vi "Pull Data For Data and Queue for DB.vi"(7 "Weather Data queue":refnum<queue>, 8 "error in (no error)":errorcluster, 9 "Airport Code":string, 10 "Time Stamp":timestamp, 11 "Refnum in":T1) -> (0 "error out":errorcluster, 3 "Refnum out":T1)   [LabVIEW 2012]
uses:
  <vilib>/httpClient/ClientHandle.ctl
  TypeDef/WeatherData.ctl
  GUI Helpers/Status Helper Action.ctl
  <vilib>/httpClient/LabVIEWHTTPClient.lvlib
panel:
  out "body":string
  out "headers":string
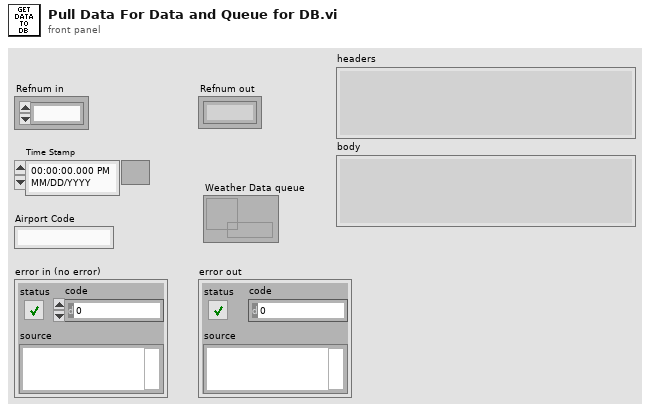
[diagram p1: front panel]
types:
  T1 = typedef "LabVIEWHTTPClient.lvlib/ClientHandle.ctl" = refnum<k1>
  T2 = typedef "Status Helper Action.ctl" = enum16{"Init", "Load Number Of Days", "Inc Add to Queue ", "Inc Get HTTP Data", "Add Push to DB", "Inc Push To DB", "Read"}
  T3 = typedef "LVDateTimeRec.ctl" = cluster{"fractional second":dbl, "second":i32, "minute":i32, "hour":i32, "day of month":i32, "month":i32, "year":i32, "day of week":i32, "day of year":i32, "DST":i32}
  T4 = typedef "WeatherData.ctl" = cluster{"TimeEST":timestamp, "TemperatureF":dbl, "DewPointF":dbl, "Humidity":i32, "Sea Level PressureIn":dbl, "VisibilityMPH":dbl, "Wind Direction":string, "Wind SpeedMPH":dbl, "Gust SpeedMPH":dbl, "PrecipitationIn":dbl, "Events":string, "Conditions":string, "WindDirDegrees":i32, "datetimeest":timestamp}
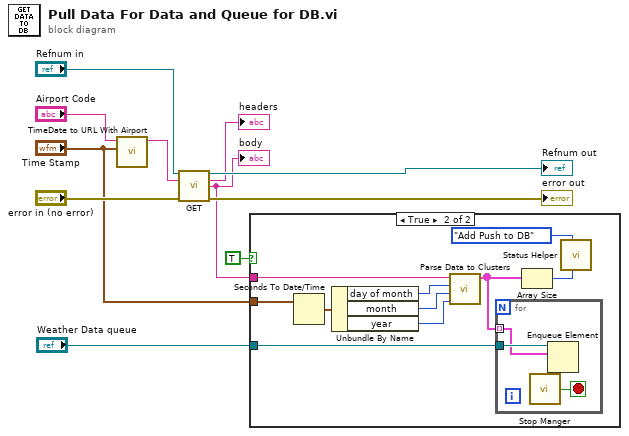
[diagram p0: block diagram]
diagram:
  n1 = call "TimeDate to URL With Airport.vi"("Time Stamp"="Time Stamp", "Airport Code"="Airport Code") -> ("URL"=w11:string)  [unwired: 9 in]
  n2 = call <vilib>:"GET.vi"("client handle"="Refnum in", "url"=w11, "error in (no error)"="error in (no error)") -> ("client handle out"=→"Refnum out":T1, "headers"=→"headers":string, "body"=w5:string, "error out"=→"error out":errorcluster)  [unwired: 9 in]
  "body" <- w5
  n3 = case shown="True" TRUE {
    tunnel: w5 -> [_ w21]
    tunnel: "Time Stamp" -> [_ w20]
    tunnel: "Weather Data queue" -> [_ w15]
    frame False {
    }
    frame True {
      n4 = Seconds To Date/Time(time stamp (now)=w20) -> (date time rec=w19:T3)  [unwired: 1 in]
      n5 = Unbundle By Name(w19) -> ("day of month"=w18:i32, "month"=w17:i32, "year"=w16:i32)
      n6 = call "Parse Data to Clusters.vi"("year"=w16, "month"=w17, "day of month"=w18, "body Text"=w21) -> ("Result Data Array"=w14:T4[])  [unwired: 7 in]
      n7 = for {
        tunnel: w15 -> [w23]
        tunnel: w14 -> [w22] mode=indexing
        stop <- w24 stop-if-true
        n8 = call "Stop Manger.vi"() -> ("Loop Stop"=w24:bool)  [unwired: 2 in]
        n9 = Enqueue Element(queue=w23, element=w22) -> ()  [unwired: 2 in, 3 out]
      }
      n10 = Array Size(array=w14) -> (size(s)=w13:i32)
      n11 = call "Status Helper"("Number of Data Pts"=w13, "Action"=Status_Helper_Action."Add Push to DB") -> ()  [unwired: 6 in, 4 out]
    }
  }
